vi "Hardware-DI-A Sim Settings-Host.vi"() -> ()   [LabVIEW 2016]
panel:
  in  "PumpCapacitance":sgl=5e-06 caption="[Farad]" format="%#_6p"
  in  "PumpInductance":sgl=0.0001 caption="[Henry]" format="%#_6p"
  in  "PumpResistance":sgl=1.0 caption="[]" format="%#_6p"
  in  "InjCapacitance":sgl=5e-06 caption="[]" format="%#_6p"
  in  "InjInductance":sgl=0.0001 caption="[]" format="%#_6p"
  in  "InjResistance":sgl=1.0 caption="[]" format="%#_6p"
  in  "SimRotations":u8=1 caption="[]"
  in  "SimSpeed":sgl=3000.0 caption="[]"
  in  "SimBatt":sgl=13.7 caption="[]"
  # "DI-A Injector and Pump Simulation \nSettings"
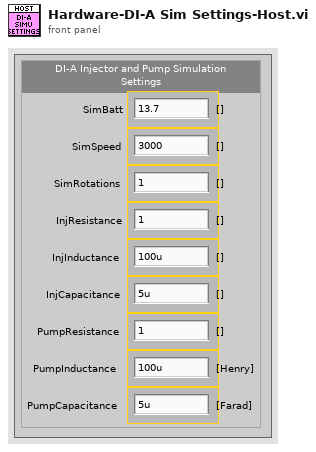
[diagram p1: front panel]
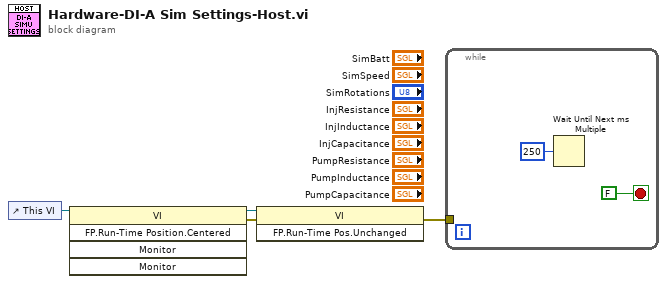
[diagram p0: block diagram]
diagram:
  n1 = control-ref of="This VI"() -> (w4:refnum<vi>)
  n2 = invoke class="VI" method="FP.Run-Time Position.Centered"(reference=w4) -> (reference out=w3:refnum<vi>, error out=w2:errorcluster)  [unwired: 4 in, 3 out]
  n3 = invoke class="VI" method="FP.Run-Time Pos.Unchanged"(reference=w3, error in=w2) -> (error out=w1:errorcluster)  [unwired: 1 in, 2 out]
  n4 = while {
    tunnel: w1 -> [_]
    stop <- FALSE stop-if-true
    n5 = Wait Until Next ms Multiple(millisecond multiple=u32 250) -> ()  [unwired: 1 out]
  }
